vi "Send Register Events to Controller.vi"(7 "Priority":T1=enum."Normal" caption="Message Priority (Normal)", 8 "error in (no error)":errorcluster, 11 "Message Enqueuer in":refnum<class "Message Enqueuer.lvclass">) -> (0 "error out":errorcluster, 3 "Message Enqueuer out":refnum<class "Message Enqueuer.lvclass">)   [LabVIEW 2023, in "MVC Actors.lvlib" / "Register Events to Controller Msg.lvclass"]
doc: "Sends the <b>MVC Actors.lvlib:Register Events to Controller Msg.lvclass</b> message.\n\nThis message will call <b>Register Events to Controller.vi</b> on the <b>MVC Actors.lvlib:View.lvclass</b> actor.\n\n<b>Register Events to Controller.vi Description</b>\nThis dynamic dispatch method has to be overridden by the child View classes to register events to the Controller."
uses:
  Register Events to Controller Msg.lvclass
  Register Events to Controller Msg.lvclass/Register Events to Controller Msg.ctl
  <vilib>/ActorFramework/Message Enqueuer/Message Enqueuer.lvclass
  C:/Program Files/National Instruments/LabVIEW 2023/vi.lib/ActorFramework/Message/Message.lvclass
  C:/Projects/Shared Libraries/Event Actors/View Messages/Register Events to Controller Msg/Register Events to Controller Msg.lvclass
  <vilib>/ActorFramework/Message Enqueuer/Message Priority.ctl
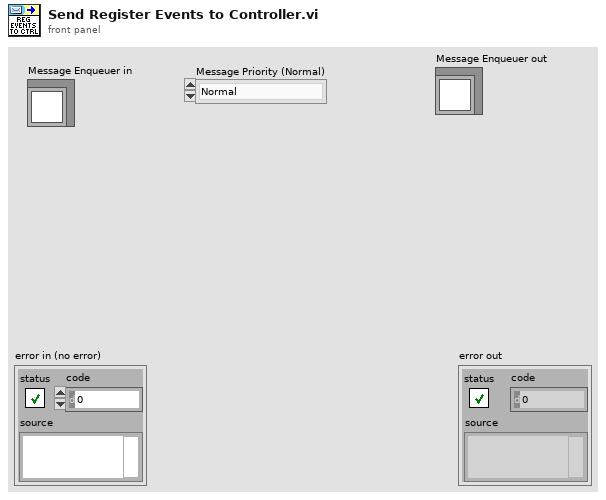
[diagram p1: front panel]
types:
  T1 = typedef "Actor Framework.lvlib/Message Enqueuer.lvclass/Message Priority.ctl" = enum16{"Low", "Normal", "High"}
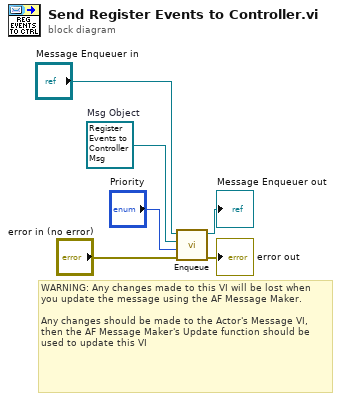
[diagram p0: block diagram]
diagram:
  w2 = refnum<class "Register Events to Controller Msg.lvclass"> refnum  # Msg Object
  # "WARNING: Any changes made to this VI will be lost when you update the message using the AF Message Maker.\n\nAny changes should be made to the Actor's Message VI, then the AF Message Maker's Update function should be used to update this VI"
  n1 = call <vilib>:"Enqueue.vi"("error in (no error)"="error in (no error)", "Message Priority (Normal)"="Priority", "Message"=w2, "Message Enqueuer in"="Message Enqueuer in") -> ("error out"=→"error out":errorcluster, "Message Enqueuer out"=→"Message Enqueuer out":refnum<class "Message Enqueuer.lvclass">)  [unwired: 6 in]
